vi "Rename State.vi"(5 "Category":string, 7 "State":string, 8 "error in (no error)":errorcluster, 9 "New State":string, 10 "New Category (\"\": Use Existing)":string, 11 "JKI SM in":refnum<class "JKI SM.lvclass">) -> (0 "error out":errorcluster, 3 "JKI SM out":refnum<class "JKI SM.lvclass">)   [LabVIEW 2013, in "JKI State Machine API.lvlib" / "JKI SM.lvclass"]
uses:
  JKI SM.lvclass
  <vilib>/Utility/traverseref.llb/TRef TravTarget.ctl
  JKI SM.lvclass/JKI SM.ctl
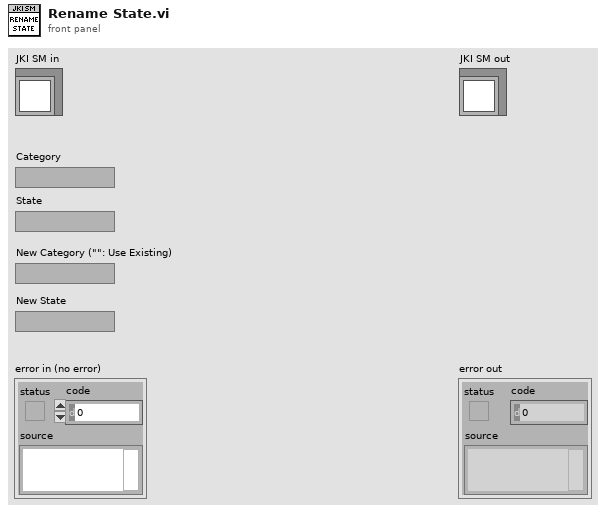
[diagram p1: front panel]
types:
  T1 = typedef "TRef TravTarget.ctl" = enum16{"FP", "BD", "Other"}
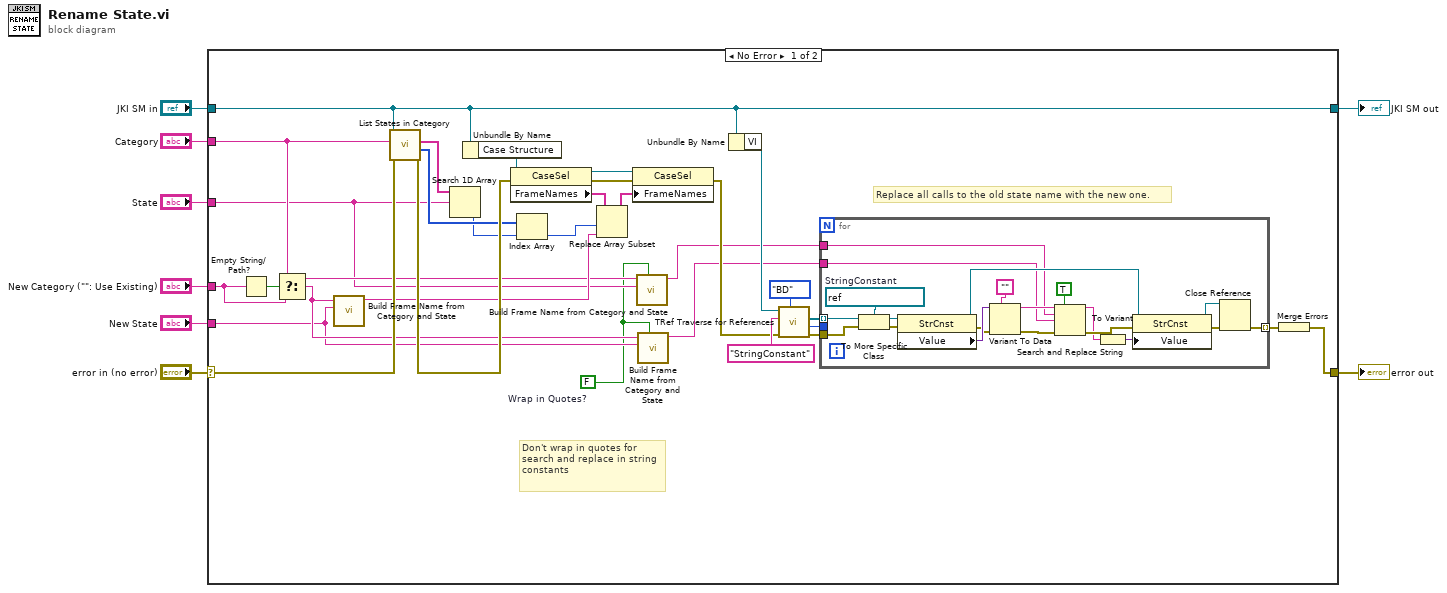
[diagram p0: block diagram]
diagram:
  n1 = case shown="No Error" "error in (no error)" {
    selector: "error in (no error)" -> [w33 w61]
    tunnel: [w23 w61] -> w7
    tunnel: [w22 w60] -> w5
    tunnel: "JKI SM in" -> [w22 w60]
    tunnel: "Category" -> [w13 _]
    tunnel: "State" -> [w12 _]
    tunnel: "New Category (\"\": Use Existing)" -> [w34 _]
    tunnel: "New State" -> [w14 _]
    frame No Error {
      w9 = FALSE  # Wrap in Quotes?
      # "Don't wrap in quotes for search and replace in string constants"
      # "Replace all calls to the old state name with the new one."
      n2 = Empty String/Path?(string/path=w34) -> (empty?=w35:bool)
      n3 = Select(t=w13, s=w35, f=w34) -> (s? t:f=w15:string)
      n4 = call "Build Frame Name from Category and State.vi"("State Name"=w14, "Category"=w15) -> ("Frame Name"=w20:string)  [unwired: 9 in]
      n5 = call "List States in Category.vi"("error in (no error)"=w33, "Category"=w13, "JKI SM in"=w22) -> ("error out"=w32:errorcluster, "State Frame Indices"=w19:i32[], "States"=w39:string[])  [unwired: 4 in, 2 out]
      n6 = Search 1D Array(1D array=w39, element=w12) -> (index of element=w18:i32)  [unwired: 1 in]
      n7 = Unbundle By Name(w22) -> ("Case Structure"=w38:refnum<vi>)
      n8 = property class="CaseSel"(reference=w38, error in=w32) -> (reference out=w37:refnum<vi>, error out=w36:errorcluster, "FrameNames"=w26:string[])
      n9 = Index Array(array=w19, index=w18) -> (element=w17:i32)
      n10 = Replace Array Subset(array=w26, new element=w20, index=w17) -> (w25:string[])
      n11 = property class="CaseSel"(reference=w37, error in=w36, "FrameNames"=w25) -> (error out=w21:errorcluster)  [unwired: 1 out]
      n12 = call "Build Frame Name from Category and State.vi"("Wrap in Quotes? (TRUE)"=w9, "State Name"=w12, "Category"=w13) -> ("Frame Name"=w11:string)  [unwired: 8 in]
      n13 = call "Build Frame Name from Category and State.vi"("Wrap in Quotes? (TRUE)"=w9, "State Name"=w14, "Category"=w15) -> ("Frame Name"=w10:string)  [unwired: 8 in]
      n14 = Unbundle By Name(w22) -> ("VI"=w31:refnum<vi>)
      n15 = call <vilib>:"TRef Traverse for References.vi"("Traverse Target"=TRef_TravTarget."BD", "error in (no error)"=w21, "Class Name"="StringConstant", "VI Refnum"=w31) -> ("error out"=w30:errorcluster, "# of Refs"=w16:i32, "References"=w29:refnum<vi>[])  [unwired: 1 in, 4 out]
      n16 = for {
        tunnel: w29 -> [w59] mode=indexing
        tunnel: w30 -> [w56]
        tunnel: w11 -> [w42]
        tunnel: w10 -> [w41]
        tunnel: [w44] -> w24 mode=indexing
        tunnel: w16 -> [_]
        w57 = refnum<vi> refnum  # StringConstant
        n17 = To More Specific Class(target class=w57, reference=w59, error in=w56) -> (specific class reference=w58:refnum<vi>, error out=w55:errorcluster)
        n18 = property class="StrCnst"(reference=w58, error in=w55) -> (reference out=w48:refnum<vi>, error out=w51:errorcluster, "Value"=w54:variant)
        n19 = Variant To Data(error in=w51, type="", Variant=w54) -> (data=w43:string, error out=w52:errorcluster)
        n20 = Search and Replace String(replace all?=TRUE ("replace all? (F)"), input string=w43, search string=w42, replace string=w41, error in=w52) -> (result string=w40:string, error out=w49:errorcluster)  [unwired: 3 in, 2 out]
        n21 = To Variant(anything=w40) -> (Variant=w47:variant)
        n22 = property class="StrCnst"(reference=w48, error in=w49, "Value"=w47) -> (reference out=w45:refnum<vi>, error out=w46:errorcluster)
        n23 = Close Reference(reference=w45, error in (no error)=w46) -> (error out=w44:errorcluster)
      }
      n24 = Merge Errors(w24) -> (w23:errorcluster)
    }
    frame Error {
    }
  }
  "error out" <- w7
  "JKI SM out" <- w5
